vi "CloseCore.vi"(8 "error in (no error)":errorcluster, 11 "MicronServer in":refnum<class "GRPCService.lvclass">) -> (0 "error out":errorcluster, 3 "MicronServer out":refnum<class "GRPCService.lvclass">)   [LabVIEW 2019, in "MicronGRPCServer.lvlib" / "GRPCService.lvclass"]
uses:
  GRPCService.lvclass
  MicronCLI/Typedefs/ServiceDetails.ctl
  GRPCService.lvclass/GRPCService.ctl
  MicronCLI/MicronCLI.lvclass
  Generated/MicronGRPCGeneratedServer/MicronGRPCGeneratedServer.lvlib
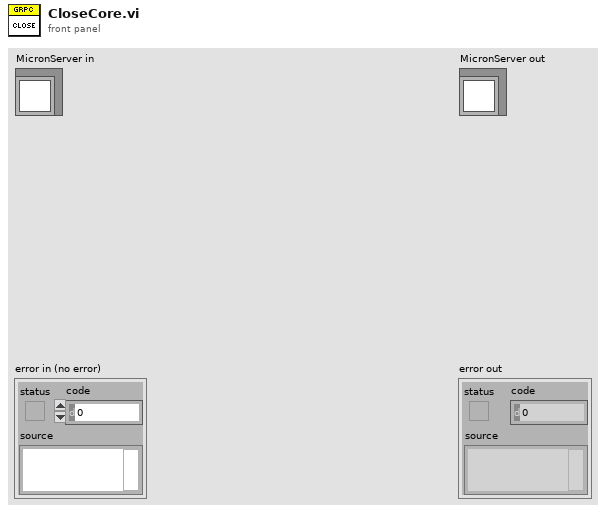
[diagram p1: front panel]
types:
  T1 = typedef "MicronCLI.lvclass/ServiceDetails.ctl" = cluster{"Network":string, "ServiceID":string}
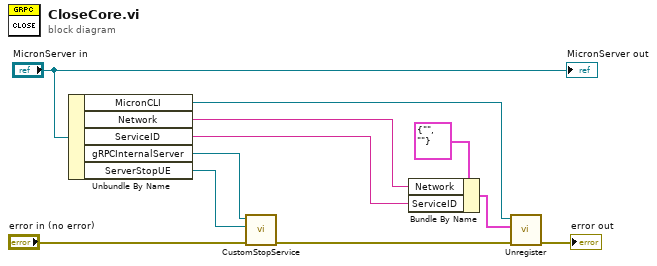
[diagram p0: block diagram]
diagram:
  n1 = Unbundle By Name("MicronServer in") -> ("MicronCLI"=w5:refnum<class "MicronCLI.lvclass">, "Network"=w3:string, "ServiceID"=w2:string, "gRPCInternalServer"=w8:refnum<class "Servicer.lvclass">, "ServerStopUE"=w7:refnum<user-event>)
  n2 = call "CustomStopService.vi"("error in (no error)"="error in (no error)", "Server Stop"=w7, "gRPC Server"=w8) -> ("error out"=w10:errorcluster)  [unwired: 8 in]
  n3 = Bundle By Name(cluster=T1 {"Network"="", "ServiceID"=""} ("Service"), "Network"=w3, "ServiceID"=w2) -> (w1:T1)
  n4 = call-dynamic "Unregister.vi"("error in (no error)"=w10, "Service"=w1, "MicronCLI in"=w5) -> ("error out"=→"error out":errorcluster)  [unwired: 7 in, 1 out]
  "MicronServer out" <- "MicronServer in"
